vi "Update Battery Indicator.vi"(0 "Battery Indicator Reference":refnum<vi>, 7 "Battery Voltage":sgl) -> ()   [LabVIEW 2011]
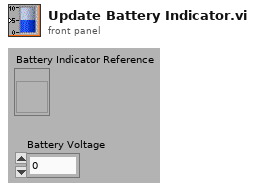
[diagram p1: front panel]
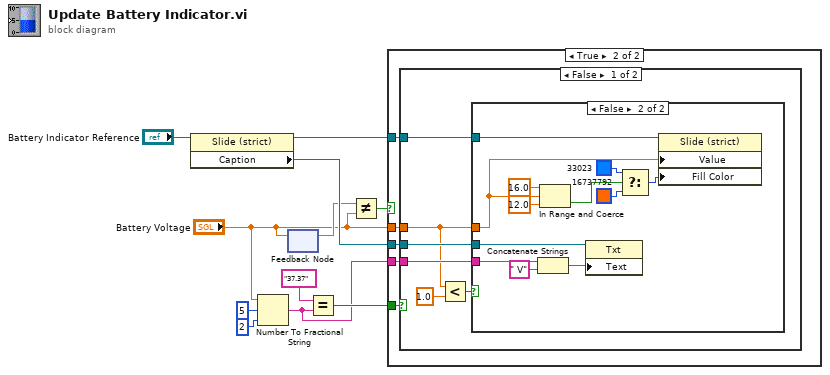
[diagram p0: block diagram]
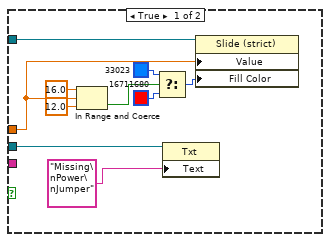
[diagram p3: hidden frame]
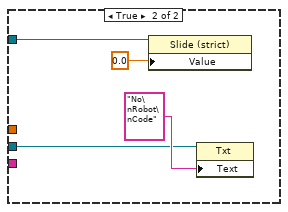
[diagram p4: hidden frame]
diagram:
  n1 = property class="Slide (strict)"(reference="Battery Indicator Reference") -> (reference out=w4:refnum<vi>, "Caption"=w5:refnum<vi>)  [unwired: 1 in, 1 out]
  n2 = Number To Fractional String(number="Battery Voltage", width (-)=i16 5, precision (6)=i16 2) -> (F-format string=w6:string)  [unwired: 1 out]
  n3 = feedback-in #1("Battery Voltage") -> ()
  n4 = feedback #1() -> (w2:sgl)  [unwired: 1 out]
  n5 = Equal?(x="37.37" ("F-format string"), y=w6) -> (x = y?=w8:bool)
  n6 = Not Equal?(x=w2, y="Battery Voltage") -> (x != y?=w3:bool)
  n7 = case shown="True" w3 {
    tunnel: w8 -> [_ w16]
    tunnel: w6 -> [_ w15]
    tunnel: w5 -> [_ w14]
    tunnel: w4 -> [_ w13]
    tunnel: "Battery Voltage" -> [_ w12]
    frame False {
    }
    frame True {
      n8 = case shown="False" w16 {
        tunnel: w12 -> [w19 _]
        tunnel: w15 -> [w22 _]
        tunnel: w13 -> [w21 w45]
        tunnel: w14 -> [w20 w47]
        frame False {
          n9 = Less?(x=w19, y=sgl 1.0 ("x")) -> (x < y?=w18:bool)
          n10 = case shown="False" w18 {
            tunnel: w22 -> [_ w44]
            tunnel: w21 -> [w32 w42]
            tunnel: w19 -> [w31 w41]
            tunnel: w20 -> [w23 w39]
            frame True {
              n11 = In Range and Coerce(upper limit=sgl 16.0, x=w31, lower limit=sgl 12.0) -> (In Range?=w27:bool)  [unwired: 1 out]
              n12 = Select(t=u32 33023, s=w27, f=u32 16711680) -> (s? t:f=w30:u32)
              n13 = property class="Txt"(reference=w23, "Text"="Missing\nPower\nJumper" ("Label.Text")) -> ()  [unwired: 1 in, 2 out]
              n14 = property class="Slide (strict)"(reference=w32, "Value"=w31, "Fill Color"=w30) -> ()  [unwired: 1 in, 2 out]
            }
            frame False {
              n15 = Concatenate Strings(w44, " V" ("string")) -> (w38:string)
              n16 = In Range and Coerce(upper limit=sgl 16.0, x=w41, lower limit=sgl 12.0) -> (In Range?=w35:bool)  [unwired: 1 out]
              n17 = property class="Txt"(reference=w39, "Text"=w38) -> ()  [unwired: 1 in, 2 out]
              n18 = Select(t=u32 33023, s=w35, f=u32 16737792) -> (s? t:f=w40:u32)
              n19 = property class="Slide (strict)"(reference=w42, "Value"=w41, "Fill Color"=w40) -> ()  [unwired: 1 in, 2 out]
            }
          }
        }
        frame True {
          n20 = property class="Slide (strict)"(reference=w45, "Value"=sgl 0.0) -> ()  [unwired: 1 in, 2 out]
          n21 = property class="Txt"(reference=w47, "Text"="No\nRobot\nCode" ("Label.Text")) -> ()  [unwired: 1 in, 2 out]
        }
      }
    }
  }
